vi "TestActuatorInterlock.vi"(3 "Input_Value_Boolean":bool, 4 "Input_Value_Double":dbl, 5 "Actuator_Name":string) -> (0 "Output_Value_Boolean":bool, 1 "Output_Value_Double":dbl, 2 "In_Test_Mode":bool)   [LabVIEW 2019]
doc: "This VI functions as an interlock, allowing operators to bypass the control logic for each actuator and test it using basic commands. This VI supports both floating point and boolean outputs. It requires integration with global variables storing the test signal and the operator's actuator selection. It is intended to integrate with the standard FRC 4265 control architecture."
uses:
  dsdata.vi
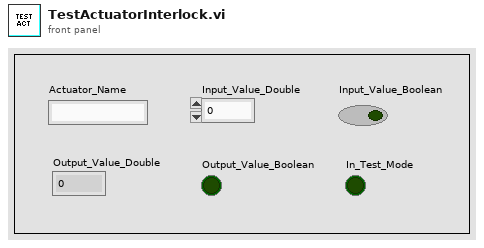
[diagram p1: front panel]
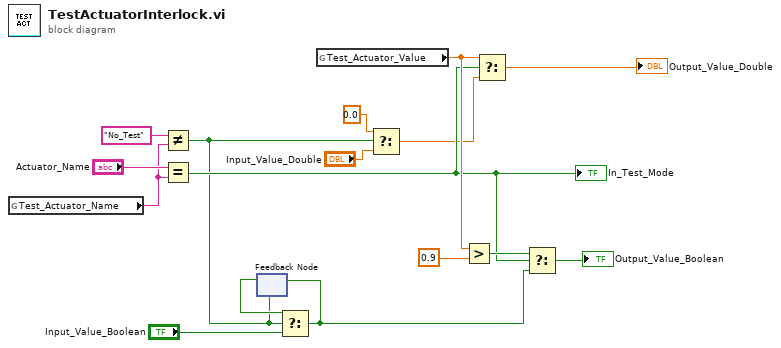
[diagram p0: block diagram]
diagram:
  n1 = global read "dsdata.vi" "Test_Actuator_Name"() -> (w1:string)
  n2 = Not Equal?(x="No_Test", y=w1) -> (x != y?=w2:bool)
  n3 = Equal?(x="Actuator_Name", y=w1) -> (x = y?=w11:bool)
  "In_Test_Mode" <- w11
  n4 = feedback #1(w2) -> (w3:bool)
  n5 = Select(t=w3, s=w2, f="Input_Value_Boolean") -> (s? t:f=w4:bool)
  n6 = feedback-in #1(w4) -> ()
  n7 = global read "dsdata.vi" "Test_Actuator_Value"() -> (w15:dbl)
  n8 = Select(t=0.0, s=w2, f="Input_Value_Double") -> (s? t:f=w6:dbl)
  n9 = Greater?(x=w15, y=0.9) -> (0:w13:bool)
  n10 = Select(t=w15, s=w11, f=w6) -> (s? t:f=→"Output_Value_Double":dbl)
  n11 = Select(t=w13, s=w11, f=w4) -> (s? t:f=→"Output_Value_Boolean":bool)
